vi "DiffDrivePoseEst_VisionCorrect_Kalman_H_Callback.vi"(9 "U":T1, 10 "X":T1, 11 "ExtraPassedData":variant) -> (0 "Error":bool, 3 "Result":T1)   [LabVIEW 2019, in "Trajectory_Library.lvlib"]
doc: "Internal function used by DiffDrivePoseEst_Update routine used by the VisionCorrect routine.\n\nInputs:\n - ExtraPassedData -- Variant of extra data used by this function. (This value is not used.)\n - X -- X matrix\n - U -- U matrix\n\nOutputs:\n - Result -- Resulting matrix\n - Error -- If TRUE, an error occured."
uses:
  Trajectory_Library.lvlib
  <vilib>/Analysis/Matrix/Datatypes/RealMatrix.ctl
  <vilib>/Analysis/Matrix/NI_Matrix.lvlib
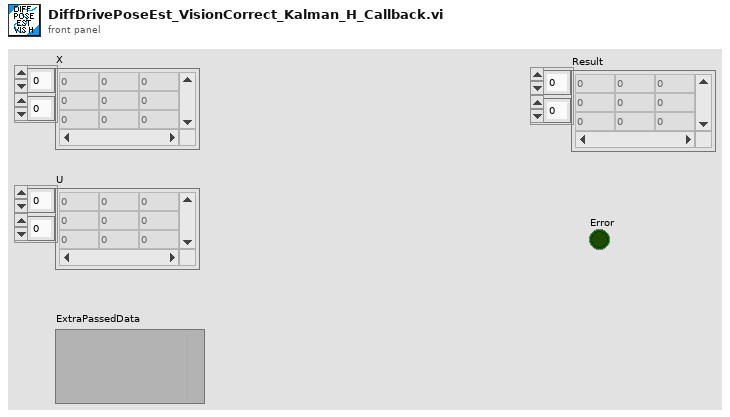
[diagram p1: front panel]
types:
  T1 = typedef "NI_Matrix.lvlib/RealMatrix.ctl" = dbl[][]
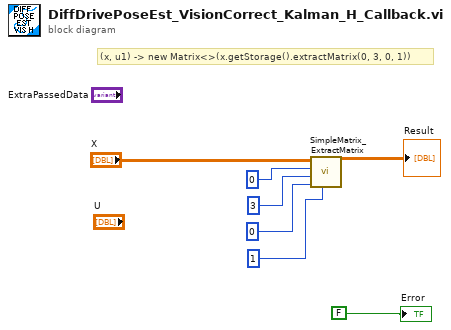
[diagram p0: block diagram]
diagram:
  # "(x, u1) -> new Matrix<>(x.getStorage().extractMatrix(0, 3, 0, 1))"
  n1 = call "SimpleMatrix_ExtractMatrix.vi"("StopColumnPlus1"=1 ("StartingColumn"), "StartingColumn"=0, "StopRowPlus1"=3, "StartingRow"=0, "input matrix"="X") -> ("output matrix"=→"Result":T1)  [unwired: 6 in]
  "Error" <- FALSE
